vi "TreadSafety.vi"(2 "%Power (10)":u8=10, 4 "Left Tread Speed":i8, 8 "Right Tread Speed":i8) -> (1 "Left Tread Speed":i8, 5 "Right Tread Speed":i8)   [LabVIEW 2010, in "Drive Trains.lvlib"]
uses:
  Drive Trains.lvlib
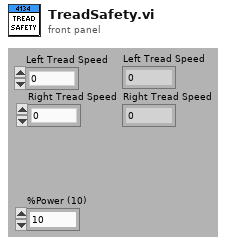
[diagram p1: front panel]
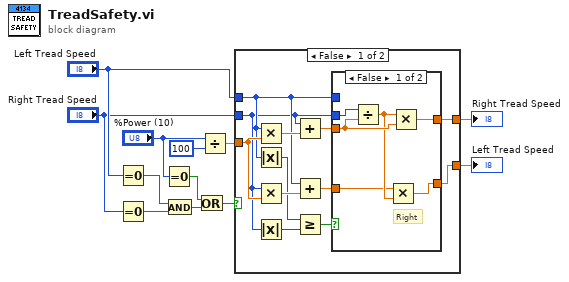
[diagram p0: block diagram]
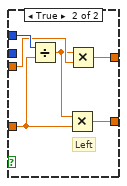
[diagram p2: hidden frame]
diagram:
  n1 = Equal To 0?(x="Left Tread Speed") -> (x = 0?=w5:bool)
  n2 = Equal To 0?(x="Right Tread Speed") -> (x = 0?=w4:bool)
  n3 = Equal To 0?(x="%Power (10)") -> (x = 0?=w6:bool)
  n4 = And(x=w5, y=w4) -> (x .and. y?=w8:bool)
  n5 = Or(x=w6, y=w8) -> (x .or. y?=w7:bool)
  n6 = Divide(x="%Power (10)", y=u8 100) -> (x/y=w3:dbl)
  n7 = case shown="False" w7 {
    tunnel: w3 -> [w24 _]
    tunnel: "Left Tread Speed" -> [w16 w38]
    tunnel: "Right Tread Speed" -> [w15 w37]
    tunnel: [w14 w38] -> w12
    tunnel: [w13 w37] -> w11
    frame False {
      n8 = Multiply(x=w16, y=w24) -> (x*y=w22:dbl)
      n9 = Absolute Value(x=w16) -> (abs(x)=w21:i8)
      n10 = Multiply(x=w15, y=w24) -> (x*y=w23:dbl)
      n11 = Absolute Value(x=w15) -> (abs(x)=w20:i8)
      n12 = Add(x=w15, y=w22) -> (x+y=w17:dbl)
      n13 = Add(x=w16, y=w23) -> (x+y=w18:dbl)
      n14 = Greater Or Equal?(x=w21, y=w20) -> (x >= y?=w19:bool)
      n15 = case shown="False" w19 {
        tunnel: w16 -> [_ w34]
        tunnel: w15 -> [w30 _]
        tunnel: w18 -> [w27 w33]
        tunnel: w17 -> [w29 w32]
        tunnel: [w25 w36] -> w13
        tunnel: [w26 w35] -> w14
        frame False {
          # "Right"
          n16 = Divide(x=w30, y=w29) -> (x/y=w28:dbl)
          n17 = Multiply(x=w27, y=w28) -> (x*y=w26:dbl)
          n18 = Multiply(x=w28, y=w29) -> (x*y=w25:dbl)
        }
        frame True {
          # "Left"
          n19 = Divide(x=w34, y=w33) -> (x/y=w31:dbl)
          n20 = Multiply(x=w31, y=w33) -> (x*y=w35:dbl)
          n21 = Multiply(x=w31, y=w32) -> (x*y=w36:dbl)
        }
      }
    }
    frame True {
    }
  }
  "Right Tread Speed" <- w11
  "Left Tread Speed" <- w12
